vi "ConnectionHeaderParse.vi"(3 "TCPROS Connection Header":string) -> (0 "Values":string[](array[string]), 1 "Fields":string[](array[string]))   [LabVIEW 2015]
doc: "Parses the TCPROS connection header and returns all found fields and their respective values"
uses:
  MessageParsing/std_msgs/subs/parse_u32_scalar.vi
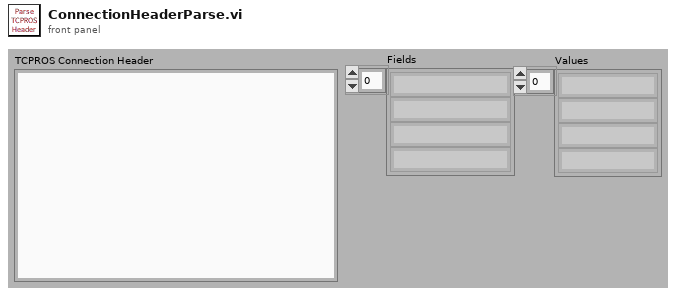
[diagram p1: front panel]
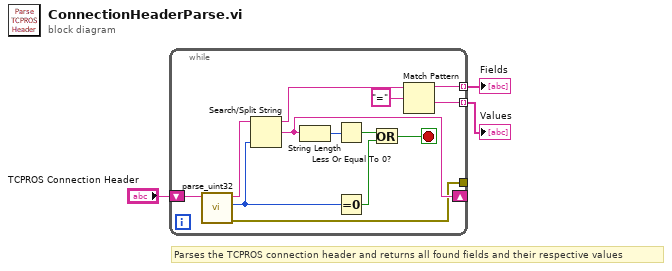
[diagram p0: block diagram]
diagram:
  # "Parses the TCPROS connection header and returns all found fields and their respective values"
  n1 = while {
    shift-right: [w13] -> _
    shift-left: "TCPROS Connection Header" -> [w15]
    tunnel: [w11] -> w2 mode=indexing
    tunnel: [w9] -> w1 mode=indexing
    tunnel: [w8] -> _
    stop <- w6 stop-if-true
    n2 = call-poly "parse_uint32.vi"("msg in"=w15) -> ("error out"=w8:errorcluster, "number"=w5:u32, "msg out"=w14:string)  [unwired: 4 in]
    n3 = Search/Split String(string=w14, offset (0)=w5) -> (substring before match=w12:string, match + rest of string=w13:string)  [unwired: 1 in, 1 out]
    n4 = String Length(string=w13) -> (length=w16:i32)
    n5 = Less Or Equal To 0?(x=w16) -> (x <= 0?=w7:bool)
    n6 = Equal To 0?(x=w5) -> (x = 0?=w4:bool)
    n7 = Or(x=w7, y=w4) -> (x .or. y?=w6:bool)
    n8 = Match Pattern(string=w12, regular expression="=") -> (before substring=w11:string, after substring=w9:string)  [unwired: 1 in, 2 out]
  }
  "Fields" <- w2
  "Values" <- w1
